vi "RichToFlatcif_waveformmonitor_WaveformEnable.vi"(5 "OutputClusterType":T1, 11 "InputCluster":T2) -> (3 "OutputCluster":T1)   [LabVIEW 2021, in "CIFWaveformMonitor_client.lvlib"]
uses:
  CIFWaveformMonitor_client.lvlib
  cif_waveformmonitor_WaveformEnable.ctl
  cif_waveformmonitor_WaveformEnable_Flat.ctl
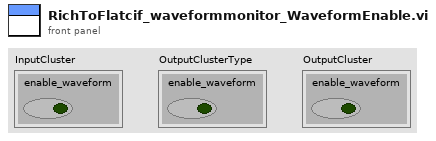
[diagram p1: front panel]
types:
  T1 = typedef "CIFWaveformMonitor_client.lvlib/cif_waveformmonitor_WaveformEnable_Flat.ctl" = cluster{"enable_waveform":bool}
  T2 = typedef "CIFWaveformMonitor_client.lvlib/cif_waveformmonitor_WaveformEnable.ctl" = cluster{"enable_waveform":bool}
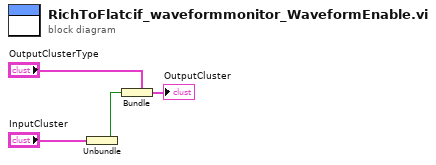
[diagram p0: block diagram]
diagram:
  n1 = Unbundle "Unbundle"("InputCluster") -> ("enable_waveform"=w1:bool)
  n2 = Bundle "Bundle"(cluster="OutputClusterType", "enable_waveform"=w1) -> (→"OutputCluster":T1)
